vi "cRIO - Set Time.vi"(10 "cRIO IP":string="192.168.1.50", 11 "shared variable RT Library":string="ni.var.psp://192.168.1.50/RT Library") -> (0 "Shared Variable":errorcluster, 1 "Set Time":errorcluster)   [LabVIEW 2013]
uses:
  <vilib>/nisyscfg/Close (System).vi
  <vilib>/nisyscfg/nisyscfg.lvlib
panel:
  in  "Set Time 2":bool
  in  "Predefined":timestamp=timestamp(3495481495 s since 1904-01-01)
  in  "Set Time":bool
  in  "Stop":bool
  out "Current":timestamp=timestamp(3472018510.6857343 s since 1904-01-01)
  out "cRIO Timestamp":timestamp=timestamp(3472018510.658165 s since 1904-01-01)
  out "detailed result":string
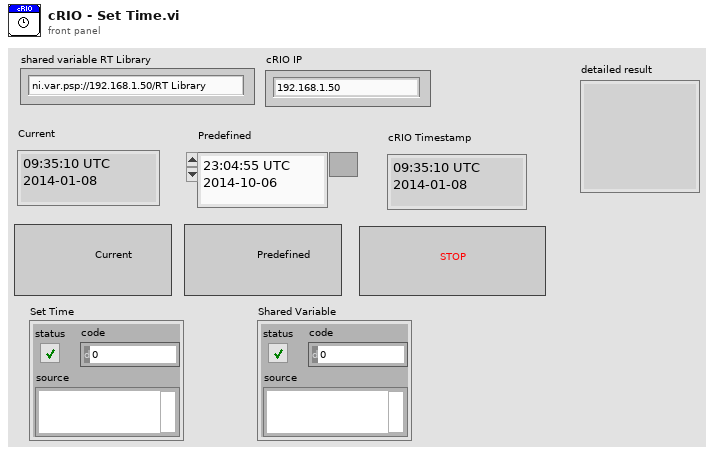
[diagram p1: front panel]
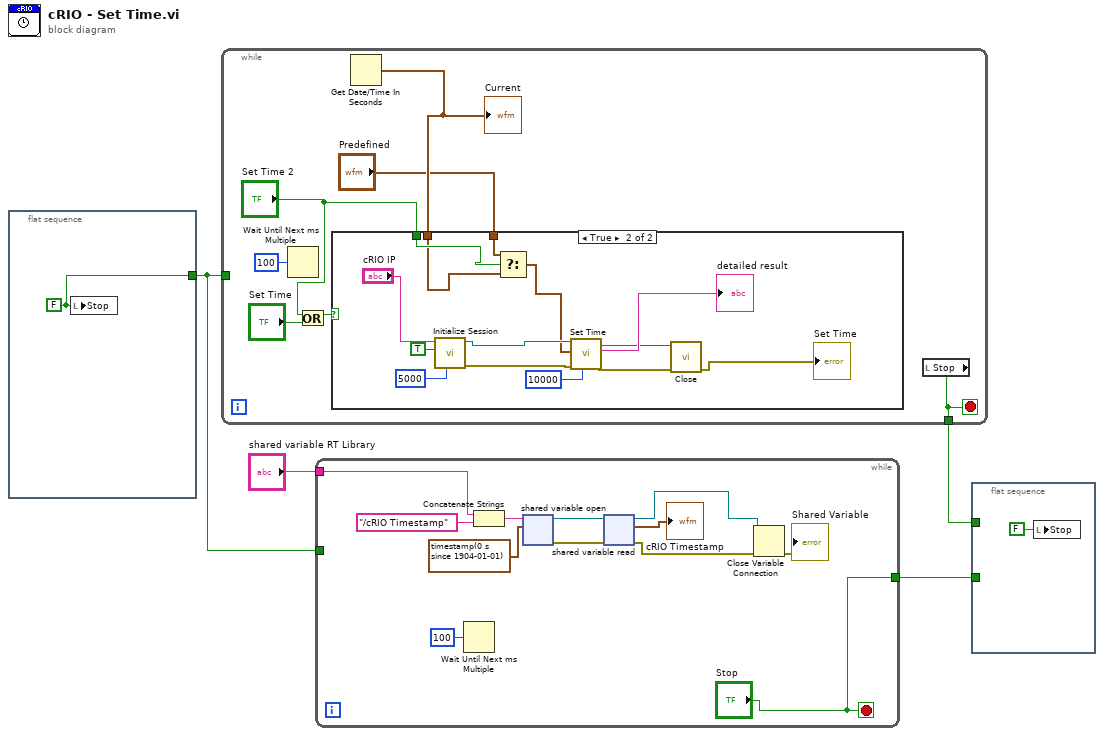
[diagram p0: block diagram]
diagram:
  n1 = flat-sequence {
    tunnel: [w5] -> w1
    frame #0 {
      w5 = FALSE ("Stop")
      n2 = local write "Stop"(w5) -> ()
    }
  }
  n3 = while {
    tunnel: [w11] -> w3
    tunnel: w1 -> [_]
    stop <- w11 stop-if-true
    n4 = Wait Until Next ms Multiple(millisecond multiple=u32 100) -> ()  [unwired: 1 out]
    n5 = Or(x="Set Time 2", y="Set Time") -> (x .or. y?=w9:bool)
    n6 = Get Date/Time In Seconds() -> (seconds since 1Jan1904=w10:timestamp)
    "Current" <- w10
    n7 = case shown="True" w9 {
      tunnel: w10 -> [_ w14]
      tunnel: "Set Time 2" -> [_ w16]
      tunnel: "Predefined" -> [_ w15]
      frame False {
      }
      frame True {
        n8 = call <vilib>:"Initialize Session.vi"("connect timeout in ms (4s)"=u32 5000, "force property refresh (T)"=TRUE, "target (localhost)"="cRIO IP") -> ("error out"=w23:errorcluster, "session out"=w24:refnum<k21>)  [unwired: 7 in]
        n9 = Select(t=w15, s=w16, f=w14) -> (s? t:f=w13:timestamp)
        n10 = call <vilib>:"Set Time.vi"("remote timeout in ms (5m)"=u32 10000, "error in (no error)"=w23, "time"=w13, "session in (localhost)"=w24) -> ("error out"=w21:errorcluster, "detailed result"=→"detailed result":string, "session out"=w22:refnum<k21>)  [unwired: 4 in, 1 out]
        n11 = call-poly <vilib>:"Close.vi"("error in (no error)"=w21, "session in"=w22) -> ("error out"=→"Set Time":errorcluster)  [unwired: 9 in]
      }
    }
    n12 = local read "Stop"() -> (w11:bool)
  }
  n13 = while {
    tunnel: "shared variable RT Library" -> [w29]
    tunnel: ["Stop"] -> w2
    tunnel: w1 -> [_]
    stop <- "Stop" stop-if-true
    n14 = Wait Until Next ms Multiple(millisecond multiple=u32 100) -> ()  [unwired: 1 out]
    n15 = Concatenate Strings(w29, "/cRIO Timestamp" ("string")) -> (w37:string)
    n16 = shared-variable-open(w37, timestamp(0 s since 1904-01-01)) -> (w34:refnum<k21>, w33:errorcluster)  [unwired: 2 in]
    n17 = shared-variable-read(w34, w33) -> (w32:refnum<k21>, w31:errorcluster, →"cRIO Timestamp":timestamp)  [unwired: 1 out]
    n18 = Close Variable Connection(8:w31, 11:w32) -> (0:→"Shared Variable":errorcluster)
  }
  n19 = flat-sequence {
    tunnel: w3 -> [_]
    tunnel: w2 -> [_]
    frame #0 {
      n20 = local write "Stop"(FALSE ("Stop")) -> ()
    }
  }
